vi "Trigger.vi"(2 "Gate Length in Seconds (-1)":dbl=-1.0, 3 "Sense":T1, 4 "Threshold":dbl format="%0.9f", 5 "Waveform":waveform(dbl)) -> (0 "Index":u32, 1 "Satisfied":bool)   [LabVIEW 2013]
uses:
  <vilib>/express/express signal manip/TriggerBlock.llb/triggerSense.ctl
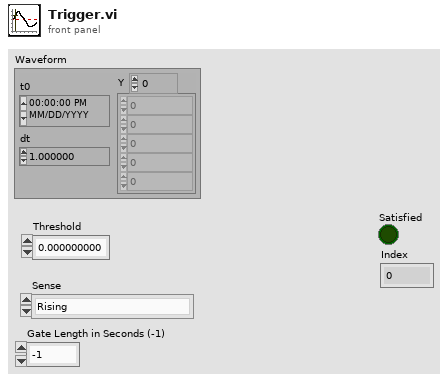
[diagram p1: front panel]
types:
  T1 = typedef "triggerSense.ctl" = enum32{"Rising", "Rising or Falling", "Falling"}
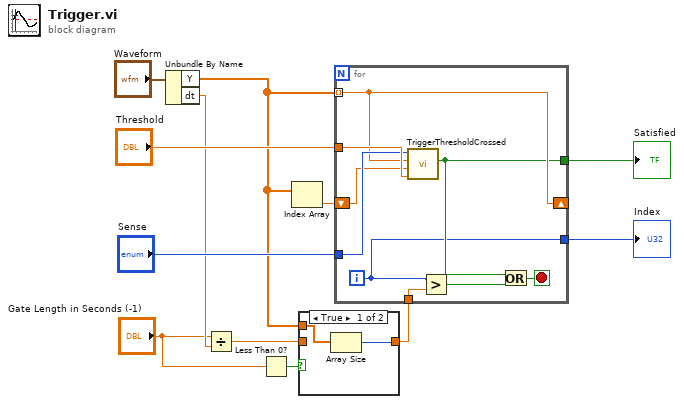
[diagram p0: block diagram]
diagram:
  n1 = Unbundle By Name("Waveform") -> ("Y"=w4:dbl[], "dt"=w6:dbl)
  n2 = Divide(x="Gate Length in Seconds (-1)", y=w6) -> (x/y=w3:dbl)
  n3 = Less Than 0?(x="Gate Length in Seconds (-1)") -> (x < 0?=w5:bool)
  n4 = Index Array(array=w4) -> (element=w10:dbl)  [unwired: 1 in]
  n5 = case shown="True" w5 {
    tunnel: w4 -> [w14 _]
    tunnel: w3 -> [_ w15]
    tunnel: [w13 w15] -> w2
    frame True {
      n6 = Array Size(array=w14) -> (size(s)=w13:i32)
    }
    frame False {
    }
  }
  n7 = for {
    tunnel: w4 -> [w22] mode=indexing
    tunnel: "Threshold" -> [w24]
    tunnel: [w19] -> w8
    tunnel: "Sense" -> [w23]
    shift-right: [w22] -> _
    shift-left: w10 -> [w21]
    tunnel: [w16] -> w9
    tunnel: w2 -> [w18]
    i -> [w16]
    stop <- w20 stop-if-true
    n8 = call "TriggerThresholdCrossed.vi"("Threshold"=w24, "Last"=w21, "Current"=w22, "Sense"=w23) -> ("Satisfied"=w19:bool)  [unwired: 7 in]
    n9 = Greater?(x=w16, y=w18) -> (0:w17:bool)
    n10 = Or(x=w19, y=w17) -> (x .or. y?=w20:bool)
  }
  "Index" <- w9
  "Satisfied" <- w8
